vi "CstEplapseTime.vi"(1 "Range":u32=2, 2 "Freq":u32=120, 3 "InitCurrentTime":u32) -> (0 "Fetch?":bool)   [LabVIEW 2015]
panel:
  in  "StartPt":u32=1
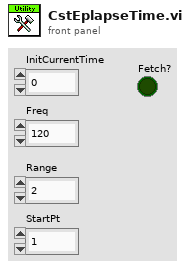
[diagram p1: front panel]
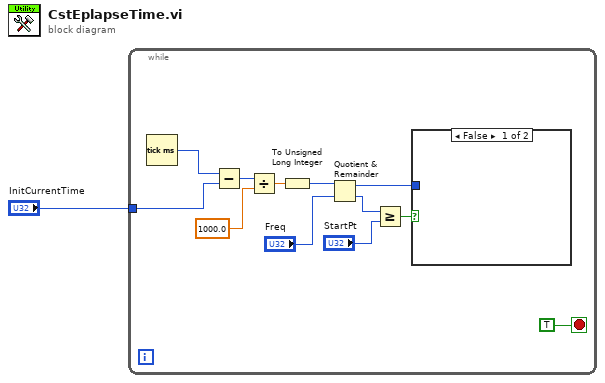
[diagram p0: block diagram]
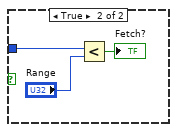
[diagram p2: hidden frame]
diagram:
  n1 = while {
    tunnel: "InitCurrentTime" -> [w11]
    stop <- TRUE stop-if-true
    n2 = Tick Count (ms)() -> (millisecond timer value=w12:u32)
    n3 = Subtract(x=w12, y=w11) -> (x-y=w5:u32)
    n4 = Divide(x=w5, y=1000.0) -> (x/y=w3:dbl)
    n5 = To Unsigned Long Integer(number=w3) -> (unsigned 32bit integer=w2:u32)
    n6 = Quotient & Remainder(x=w2, y="Freq") -> (x-y*floor(x/y)=w10:u32, floor(x/y)=w7:u32)
    n7 = Greater Or Equal?(x=w7, y="StartPt") -> (x >= y?=w8:bool)
    n8 = case shown="False" w8 {
      tunnel: w10 -> [_ w16]
      frame False {
      }
      frame True {
        n9 = Less?(x=w16, y="Range") -> (x < y?=→"Fetch?":bool)
      }
    }
  }
